vi "Read From Spreadsheet File2.vi"(4 "array conversion":u16(ring) items=["standard tab", " arrbitrary spaces"], 6 "transpose (no:F)":bool, 7 "format (%.3f)":string="%.3f", 8 "max characters/row  (no limit:0)":i32, 9 "start of read offset (chars.:0 )":i32, 10 "number of rows (all:-1)":i32=-1, 11 "file path (dialog if empty)":path) -> (0 "EOF?":bool, 1 "mark after read (chars.)":i32, 2 "first row":sgl[](array[numeric]) format="%.3f", 3 "all rows":sgl[][](array[numeric]) format="%.4f", 5 "new file path (Not A Path if cancelled)":path)   [LabVIEW 2018]
doc: "Reads a specified number of lines or rows from a numeric text file beginning at a specified character offset and converts the data to a 2D single-precision array of numbers. You can optionally transpose the array. The VI opens the file beforehand and closes it afterwards. You can use this VI to read spreadsheet file saved in text format that have columns separated with tab characters and rows terminated with EOL characters. See the note on the diagram if your file has other separators or terminators.\n\nfile path is the path name of the file. If file path is empty (default value) or is Not A Path, the VI displays a File dialog box from which you can select a file. Error 43 occurs if the user cancels the dialog. \n\nnumber of rows is the maximum number of rows or lines the VI reads. The default value is -1 rows, which means to read the entire file. For this VI, a row is a character string ending with a carriage return, line feed, or a carriage return followed by a line feed; a string ending at the EOF; or a string that has the maximum line length specified by the max characters per row input.\n\nstart of read offset is the position in the file, measured in characters (or bytes), at which the VI begins reading.\n\nmax characters per row is the maximum number of characters the VI reads before ending the search for the end of a row or line. The default is 0, which means that there is no limit to the number of characters the VI reads.\n\ntranspose? Set TRUE to transpose the data after converting it from a string. The default value is FALSE.\n\nformat specifies how to convert the characters to numbers; the default is %.3f. Refer to the discussion of format strings and the Spreadsheet String To Array function in Chapter 6, String Functions, of the LabVIEW Function Reference Manual.\n\nnew file path is the path of the file from which the VI read data. You can use this output to determine the path of a file that you open using dialog. new file path returns Not A Path if the user selects Cancel from the dialog box.\n\nall rows is the data read from the file in the form of a 2D array of single-precision numbers.\n\nfirst row is the first row of the all rows array in the form of a 1D array of single-precision numbers. You can use this output when you want to read one row into a 1D array.\n\nmark after read is the location of the file mark after the read; it points to the character in the file following the last character read.\n\nEOF? is TRUE if you attempt to read past the end of file."
panel:
  out "?":string
  in  "type (empty)":sgl[][](array[numeric]) format="%.2f"
  # "row\ncolumn"
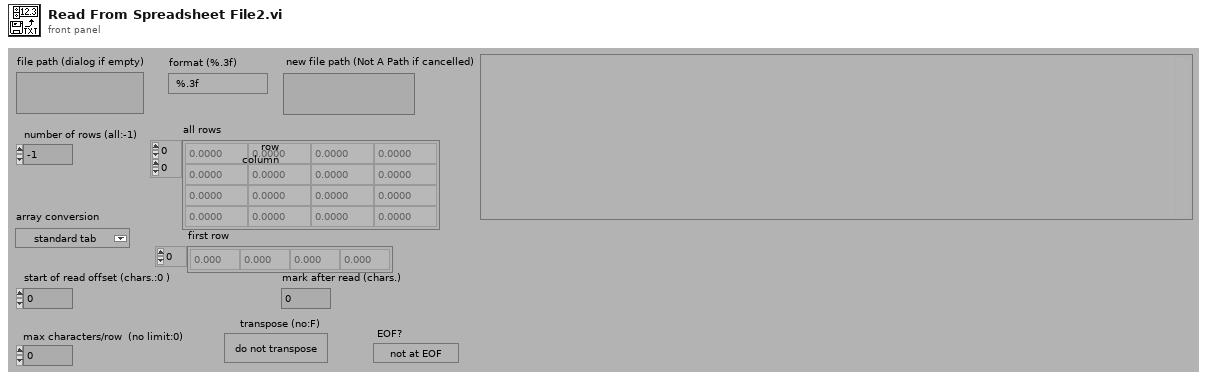
[diagram p1: front panel]
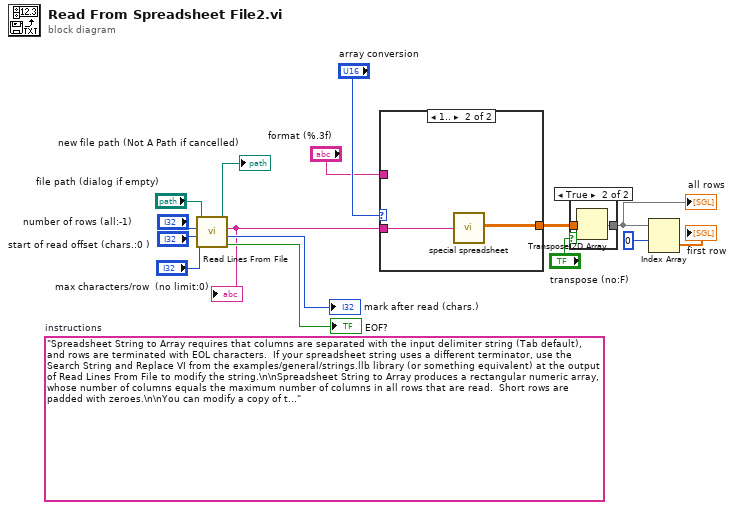
[diagram p0: block diagram]
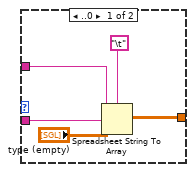
[diagram p2: hidden frame]
diagram:
  (unwired) "Spreadsheet String to Array requires that columns are separated with the input delimiter string (Tab default), and rows are terminated with EOL characters.  If your spreadsheet string uses a different terminator, use the Search String and Replace VI from the examples/general/strings.llb library (or something equivalent) at the output of Read Lines From File to modify the string.\n\nSpreadsheet String to Array produces a rectangular numeric array, whose number of columns equals the maximum number of columns in all rows that are read.  Short rows are padded with zeroes.\n\nYou can modify a copy of this VI to return the file contents into arrays of strings by changing all rows, first row, and type (empty) arrays to string arrays and by setting the format to %s."  # instructions
  n1 = call <vilib>:"Read Lines From File.vi"("file path (dialog if empty)"="file path (dialog if empty)", "number of lines (all:-1)"="number of rows (all:-1)", "start of read offset (chars.:0)"="start of read offset (chars.:0 )", "[max characters per line]  (no limit:0)"="max characters/row  (no limit:0)") -> ("new file path (Not A Path if cancelled)"=→"new file path (Not A Path if cancelled)":path, "line string"=w2:string, "mark after read (chars.)"=→"mark after read (chars.)":i32, "EOF?"=→"EOF?":bool)  [unwired: 2 in]
  "?" <- w2
  n2 = case shown="1.." "array conversion" {
    tunnel: w2 -> [w20 w21]
    tunnel: "format (%.3f)" -> [w18 _]
    tunnel: [w16 w22] -> w3
    frame ..0 {
      n3 = Spreadsheet String To Array(delimiter (Tab)="\t", format string=w18, spreadsheet string=w20, array type (2D Dbl)="type (empty)") -> (array=w16:sgl[][])
    }
    frame 1.. {
      n4 = call "special spreadsheet.vi"("input string"=w21) -> ("array"=w22:dbl[][])
    }
  }
  n5 = case shown="True" "transpose (no:F)" {
    tunnel: [w23 w25] -> w7
    tunnel: w3 -> [w23 w24]
    frame False {
    }
    frame True {
      n6 = Transpose 2D Array(2D array=w24) -> (transposed array=w25:dbl[][])
    }
  }
  "all rows" <- w7
  n7 = Index Array(array=w7, index (row)=0) -> (element=→"first row":dbl[])  [unwired: 1 in]
